vi "Cascade Wfm List.vi"(8 "error in (no error)":errorcluster, 9 "Channel Name":string, 10 "Trim and Resample Settings":cluster{"Duration":dbl, "Sample Rate":dbl}={"Duration"=0.002, "Sample Rate"=0.0} {"Sample Rate" format="%#_6pHz"; "Duration" format="%#_6ps"}, 11 "Canvas Wfm Array In":waveform(dbl)[](array[waveform])) -> (0 "error out":errorcluster, 2 "Final Flatten Wfm Channel":waveform(dbl), 3 "Canvas Wfm Array Out":waveform(dbl)[](array[waveform]))   [LabVIEW 2025, in "TDMS Waveform Creator UI.lvlib"]
uses:
  TDMS Waveform Creator UI.lvlib
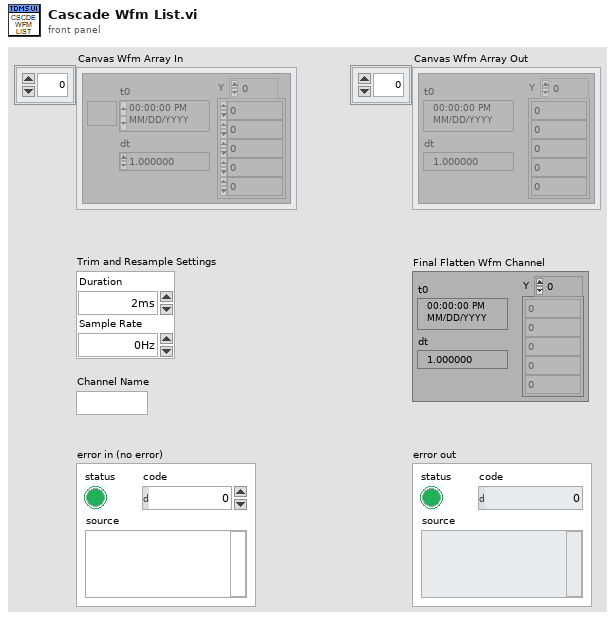
[diagram p1: front panel]
types:
  T1 = cluster{"Trim and Resample Settings":cluster{"Duration":dbl, "Sample Rate":dbl}, "Wfms Json":string[]}
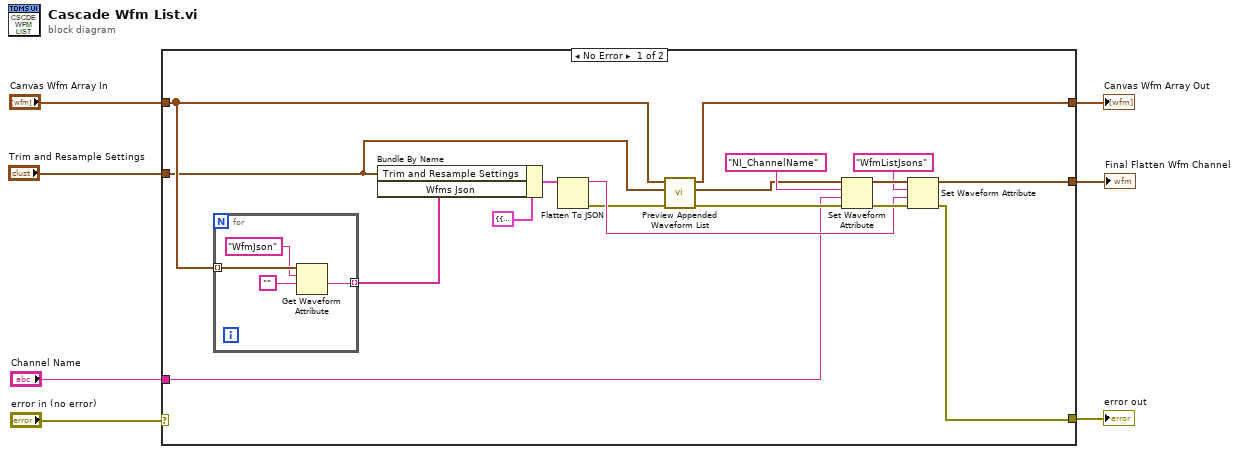
[diagram p0: block diagram]
diagram:
  n1 = case shown="No Error" "error in (no error)" {
    selector: "error in (no error)" -> [_ w30]
    tunnel: "Canvas Wfm Array In" -> [w15 w29]
    tunnel: [w14 w29] -> w5
    tunnel: "Trim and Resample Settings" -> [w11 _]
    tunnel: [w9 w30] -> w3
    tunnel: [w10 _] -> w2
    tunnel: "Channel Name" -> [w8 _]
    frame No Error {
      n2 = for {
        tunnel: w15 -> [w28] mode=indexing
        tunnel: [w25] -> w24 mode=indexing
        n3 = Get Waveform Attribute(5:"", 6:"WfmJson" ("name"), 7:w28) -> (1:w25:string)  [unwired: 1 in, 3 out]
      }
      n4 = Bundle By Name(cluster=T1 {"Trim and Resample Settings"={"Duration"=0.0, "Sample Rate"=0.0}, "Wfms Json"=[]} ("Wfm Summary"), "Trim and Resample Settings"=w11, "Wfms Json"=w24) -> (w22:T1)
      n5 = Flatten To JSON(anything=w22) -> (JSON string=w13:string, 11:w12:errorcluster)  [unwired: 2 in]
      n6 = call "Preview Appended Waveform List.vi"("error in (no error)"=w12, "Trim and Resample Settings"=w11, "Canvas Wfm Array In"=w15) -> ("error out"=w18:errorcluster, "Final Waveform"=w20:waveform(dbl), "Canvas Wfm Array Out"=w14:waveform(dbl)[])  [unwired: 6 in]
      n7 = Set Waveform Attribute(4:w18, 5:w8, 6:"NI_ChannelName" ("name"), 7:w20) -> (0:w19:errorcluster, 3:w17:waveform(dbl))  [unwired: 1 out]
      n8 = Set Waveform Attribute(4:w19, 5:w13, 6:"WfmListJsons" ("name"), 7:w17) -> (0:w9:errorcluster, 3:w10:waveform(dbl))  [unwired: 1 out]
    }
    frame Error {
    }
  }
  "error out" <- w3
  "Canvas Wfm Array Out" <- w5
  "Final Flatten Wfm Channel" <- w2
